vi "PosnMove.vi"(7 "targetPosn":i32, 8 "error in (no error)":errorcluster, 9 "isAbsolute":bool, 10 "addDwell":bool, 11 "Axis in":refnum<class "Axis.lvclass">) -> (0 "error out":errorcluster, 3 "Axis out":refnum<class "Axis.lvclass">)   [LabVIEW 2020, in "Axis.lvclass"]
uses:
  Axis.lvclass
  Axis.lvclass/Axis.ctl
  C:/Users/Jonathan/Documents/Clearpath SDK/CSharp Examples/CLRWrapper/x64/Debug/CLRWrapper.dll
  CSharp Examples/CLRWrapper/x64/Debug/CLRWrapper.dll
panel:
  out "scaledPosn":i64
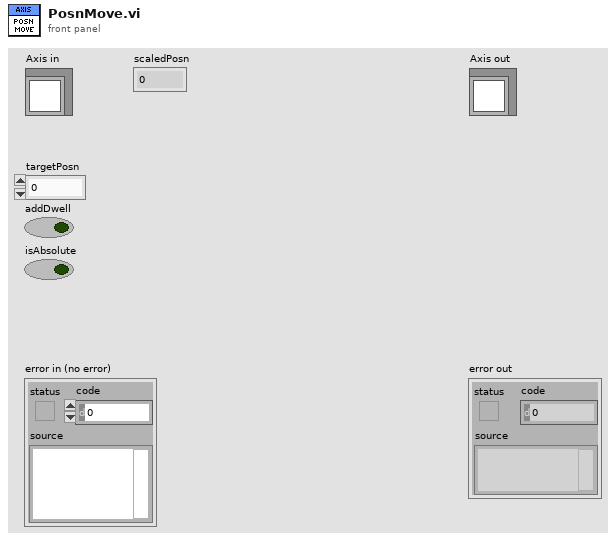
[diagram p1: front panel]
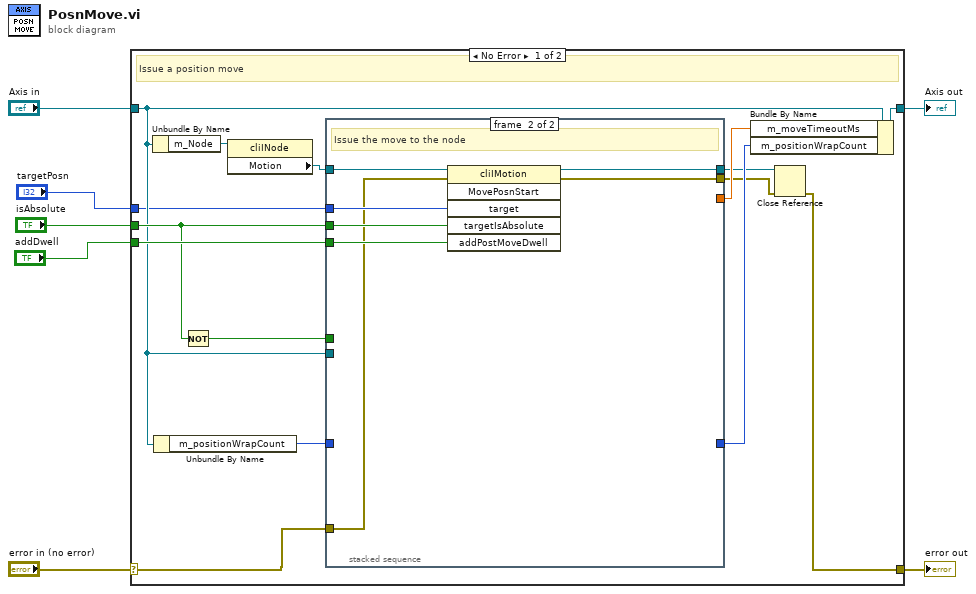
[diagram p0: block diagram]
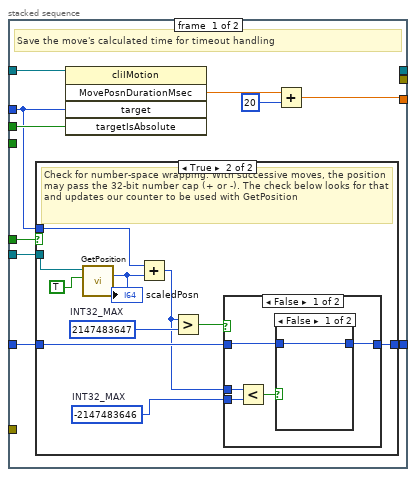
[diagram p2: hidden frame]
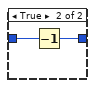
[diagram p4: hidden frame]
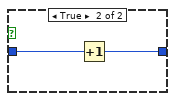
[diagram p5: hidden frame]
diagram:
  n1 = case shown="No Error" "error in (no error)" {
    selector: "error in (no error)" -> [w12 w62]
    tunnel: [w8 w62] -> w6
    tunnel: [w20 w61] -> w4
    tunnel: "Axis in" -> [w16 w61]
    tunnel: "targetPosn" -> [w15 _]
    tunnel: "isAbsolute" -> [w17 _]
    tunnel: "addDwell" -> [w21 _]
    frame No Error {
      # "Issue a position move"
      n2 = Unbundle By Name(w16) -> ("m_Node"=w11:refnum<k24>)
      n3 = Unbundle By Name(w16) -> ("m_positionWrapCount"=w14:i64)
      n4 = Not(x=w17) -> (.not. x?=w18:bool)
      n5 = property class="cliINode"(reference=w11) -> ("Motion"=w22:refnum<k24>)  [unwired: 1 in, 2 out]
      n6 = stacked-sequence {
        tunnel: w22 -> [w32 w60]
        tunnel: w21 -> [_ w57]
        tunnel: [w29 _] -> w19
        tunnel: w18 -> [w28 _]
        tunnel: w17 -> [w27 w58]
        tunnel: w16 -> [w26 _]
        tunnel: w15 -> [w25 w59]
        tunnel: w14 -> [w24 _]
        tunnel: [w23 _] -> w13
        tunnel: w12 -> [_ w56]
        tunnel: [_ w55] -> w10
        tunnel: [_ w54] -> w9
        frame #0 {
          # "Save the move's calculated time for timeout handling"
          n7 = case shown="True" w28 {
            tunnel: w26 -> [_ w43]
            tunnel: w25 -> [_ w39]
            tunnel: w24 -> [w33 w37]
            tunnel: [w33 w36] -> w23
            frame False {
            }
            frame True {
              w34 = -2147483646  # INT32_MAX
              w41 = 2147483647  # INT32_MAX
              # "Check for number-space wrapping. With successive moves, the position may\tpass the 32-bit number cap (+ or -). The check below looks for that and updates our counter to be used with GetPosition"
              n8 = call "GetPosition.vi"("includeWraps"=TRUE, "Axis in"=w43) -> ("scaledPosn"=w40:i64)  [unwired: 5 in, 4 out]
              "scaledPosn" <- w40
              n9 = Add(x=w39, y=w40) -> (x+y=w35:i64)
              n10 = Greater?(x=w35, y=w41) -> (0:w38:bool)
              n11 = case shown="False" w38 {
                tunnel: w37 -> [w45 w53]
                tunnel: [w44 w52] -> w36
                tunnel: w35 -> [w48 _]
                tunnel: w34 -> [w47 _]
                frame False {
                  n12 = Less?(x=w48, y=w47) -> (x < y?=w46:bool)
                  n13 = case shown="False" w46 {
                    tunnel: w45 -> [w49 w51]
                    tunnel: [w49 w50] -> w44
                    frame False {
                    }
                    frame True {
                      n14 = Decrement(x=w51) -> (x-1=w50:i64)
                    }
                  }
                }
                frame True {
                  n15 = Increment(x=w53) -> (x+1=w52:i64)
                }
              }
            }
          }
          n16 = invoke class="cliIMotion" method="MovePosnDurationMsec"(reference=w32, "target"=w25, "targetIsAbsolute"=w27) -> ("MovePosnDurationMsec"=w31:dbl)  [unwired: 2 in, 4 out]
          n17 = Add(x=w31, y=u64 20) -> (x+y=w29:dbl)
        }
        frame #1 {
          # "Issue the move to the node"
          n18 = invoke class="cliIMotion" method="MovePosnStart"(reference=w60, error in=w56, "target"=w59, "targetIsAbsolute"=w58, "addPostMoveDwell"=w57) -> (reference out=w54:refnum<k24>, error out=w55:errorcluster)  [unwired: 1 in, 4 out]
        }
      }
      n19 = Bundle By Name(cluster=w16, "m_moveTimeoutMs"=w19, "m_positionWrapCount"=w13) -> (w20:refnum<class "Axis.lvclass">)
      n20 = Close Reference(reference=w9, error in (no error)=w10) -> (error out=w8:errorcluster)
    }
    frame Error {
    }
  }
  "error out" <- w6
  "Axis out" <- w4
